vi "IP_地址校验IPV4.vi"(11 "IP Address":string) -> (2 "合法？":bool, 3 "所有匹配":string)   [LabVIEW 2018]
uses:
  <vilib>/regexp/Match Regular Expression.xnode
panel:
  out "匹配之后":string
  out "匹配之前":string
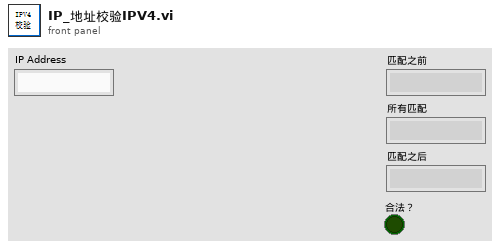
[diagram p1: front panel]
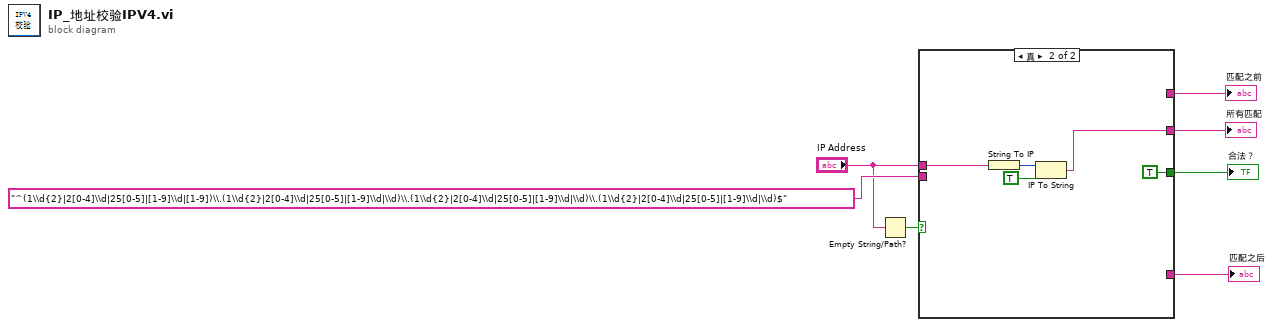
[diagram p0: block diagram]
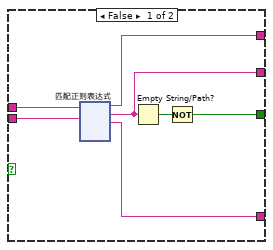
[diagram p2: hidden frame]
diagram:
  n1 = Empty String/Path?(string/path="IP Address") -> (empty?=w1:bool)
  n2 = case shown="真" w1 {
    tunnel: "^(1\\d{2}|2[0-4]\\d|25[0-5]|[1-9]\\d|[1-9])\\.(1\\d{2}|2[0-4]\\d|25[0-5]|[1-9]\\d|\\d)\\.(1\\d{2}|2[0-4]\\d|25[0-5]|[1-9]\\d|\\d)\\.(1\\d{2}|2[0-4]\\d|25[0-5]|[1-9]\\d|\\d)$" ("正则表达式") -> [w14 _]
    tunnel: "IP Address" -> [w13 w133]
    tunnel: [w12 _] -> w6
    tunnel: [w11 _] -> w5
    tunnel: [w10 w130] -> w4
    tunnel: [w8 TRUE] -> w3
    frame False {
      n3 = xnode "匹配正则表达式"("输入字符串"=w13, "正则表达式"=w14) -> ("匹配之前"=w12:string, "所有匹配"=w10:string, "匹配之后"=w11:string)  [unwired: 4 in, 2 out]
      n4 = Empty String/Path?(string/path=w10) -> (empty?=w9:bool)
      n5 = Not(x=w9) -> (.not. x?=w8:bool)
    }
    frame True {
      n6 = String To IP(1:w133) -> (0:w132:u32)
      n7 = IP To String(1:TRUE ("句点符号？(F)"), 2:w132) -> (0:w130:string)
    }
  }
  "匹配之前" <- w6
  "所有匹配" <- w4
  "匹配之后" <- w5
  "合法？" <- w3
